vi "Read.Data.vi"(5 "length":i32=-1, 7 "index":i32, 8 "error in (no error)":errorcluster, 10 "timeout ms":i32, 11 "Ref":T1) -> (0 "error out":errorcluster, 1 "Timeout?":bool, 2 "Values":dbl[](array[numeric]))   [LabVIEW 2027, in "Data Access Engine.lvlib" / "Data Access Engine.lvclass"]
uses:
  Data Access Engine.lvclass
  Types/Read.DVR.ctl
  Access Type Classes/Read/Read.lvclass
  Access Type Classes/Read/Read.lvclass/Read.ctl
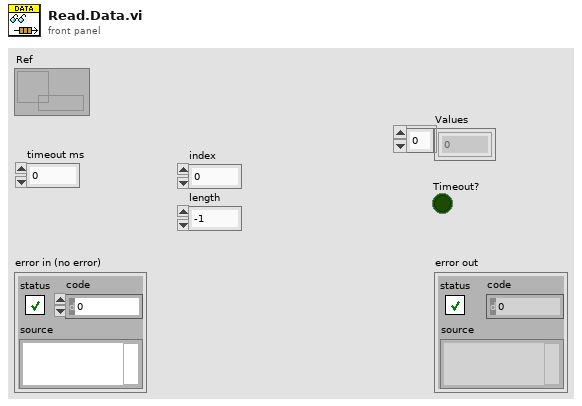
[diagram p1: front panel]
types:
  T1 = typedef "Data Access Engine.lvlib/Data Access Engine.lvclass/Read.DVR.ctl" = refnum<data-value>
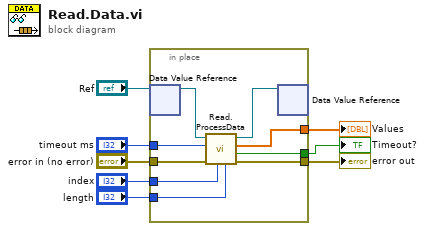
[diagram p0: block diagram]
diagram:
  n1 = in-place {
    in-place-border: "error in (no error)" -> [w17]
    in-place-border: [w16] -> w7
    in-place-border: [w13] -> w5
    in-place-border: "timeout ms" -> [w12]
    in-place-border: [w11] -> w3
    in-place-border: "index" -> [w10]
    in-place-border: "length" -> [w9]
    n2 = in-place-dvr #1("Ref") -> (w15:refnum<class "Read.lvclass">)  [unwired: 1 out]
    n3 = call "Read.ProcessData.vi"("length"=w9, "index"=w10, "error in (no error)"=w17, "timeout ms"=w12, "Read in"=w15) -> ("error out"=w16:errorcluster, "Timeout?"=w11:bool, "Data"=w13:dbl[], "Read out"=w14:refnum<class "Read.lvclass">)  [unwired: 3 in]
    n4 = in-place-dvr #1(w14) -> ()  [unwired: 2 out]
  }
  "error out" <- w7
  "Values" <- w5
  "Timeout?" <- w3
